vi "Permanent Settings.vi"(11 "Settings in in":T1) -> (3 "Settings out":T1)   [LabVIEW 2013, in "AvaSpec.lvlib" / "AvaSpec Settings.lvlib"]
uses:
  AvaSpec Settings.lvlib
  Settings.ctl
  Acquisition/Hardware Configuration.ctl
  Libraries/AS-5216-DLL/AVS settings.ctl
  Acquisition/Sphere Indicator.ctl
  Measurement Type.ctl
  Logging/Logging Configuration.ctl
  AvaSpec.lvlib
  Acquisition/AvaSpec Acquisition.lvlib
  Logging/AvaSpec Logging.lvlib
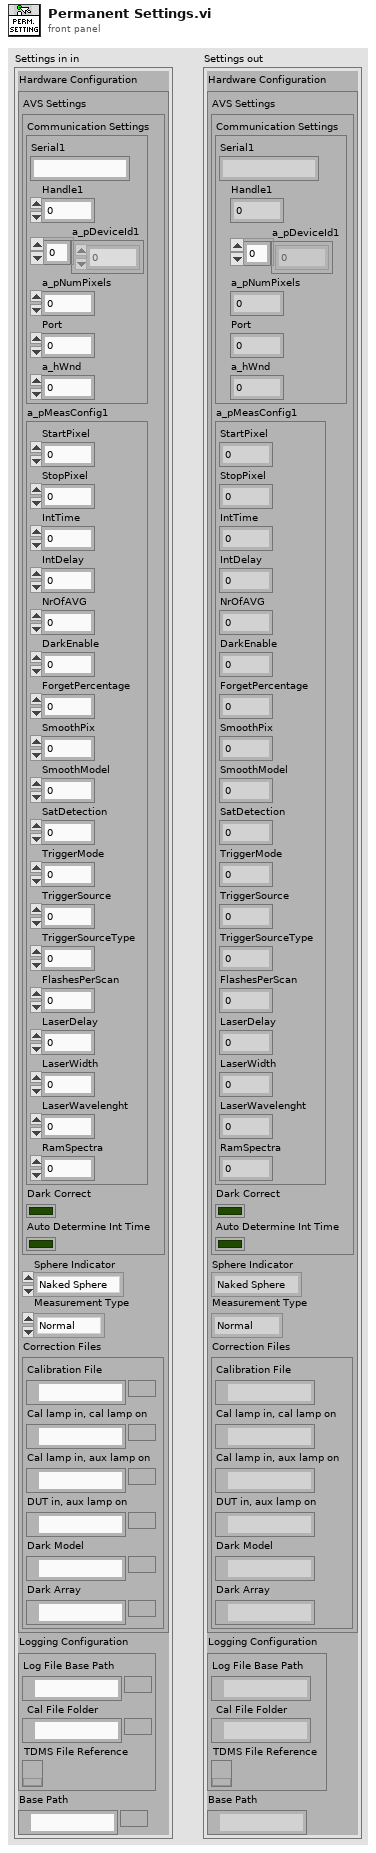
[diagram p1: front panel]
types:
  T1 = typedef "AvaSpec.lvlib/AvaSpec Settings.lvlib/Settings.ctl" = cluster{"Hardware Configuration":T2, "Logging Configuration":T6, "Base Path":path}
  T2 = typedef "AvaSpec.lvlib/AvaSpec Acquisition.lvlib/Hardware Configuration.ctl" = cluster{"AVS Settings":T3, "Sphere Indicator":T4, "Measurement Type":T5, "Correction Files":cluster{"Calibration File":path, "Cal lamp in, cal lamp on":path, "Cal lamp in, aux lamp on":path, "DUT in, aux lamp on":path, "Dark Model":path, "Dark Array":path}}
  T3 = typedef "AvaSpec.lvlib/AVS settings.ctl" = cluster{"Communication Settings":cluster{"Serial1":string, "Handle1":i32, "a_pDeviceId1":u8[], "a_pNumPixels":u16, "Port":i32, "a_hWnd":i32}, "a_pMeasConfig1":cluster{"StartPixel":u16, "StopPixel":u16, "IntTime":sgl, "IntDelay":u32, "NrOfAVG":u32, "DarkEnable":u8, "ForgetPercentage":u8, "SmoothPix":u16, "SmoothModel":u8, "SatDetection":u8, "TriggerMode":u8, "TriggerSource":u8, "TriggerSourceType":u8, "FlashesPerScan":u16, "LaserDelay":u32, "LaserWidth":u32, "LaserWavelenght":sgl, "RamSpectra":u16}, "Dark Correct":bool, "Auto Determine Int Time":bool}
  T4 = typedef "AvaSpec.lvlib/Sphere Indicator.ctl" = enum16{"Naked Sphere", "Insulated Sphere"}
  T5 = typedef "AvaSpec.lvlib/AvaSpec Acquisition.lvlib/Measurement Type.ctl" = enum16{"Normal", "Calibration", "Dark"}
  T6 = typedef "AvaSpec.lvlib/AvaSpec Logging.lvlib/Logging Configuration.ctl" = cluster{"Log File Base Path":path, "Cal File Folder":path, "TDMS File Reference":refnum<k34>}
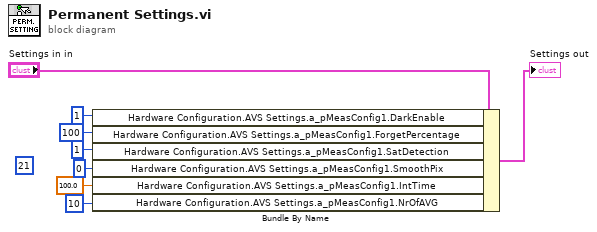
[diagram p0: block diagram]
diagram:
  (unwired) u8 21 ("Hardware Configuration.AVS Settings.a_pMeasConfig1.SmoothModel")
  n1 = Bundle By Name(cluster="Settings in in", "Hardware Configuration.AVS Settings.a_pMeasConfig1.DarkEnable"=u8 1 ("Hardware Configuration.a_pMeasConfig1.DarkEnable"), "Hardware Configuration.AVS Settings.a_pMeasConfig1.ForgetPercentage"=u8 100 ("Hardware Configuration.a_pMeasConfig1.SatDetection"), "Hardware Configuration.AVS Settings.a_pMeasConfig1.SatDetection"=u8 1 ("Hardware Configuration.a_pMeasConfig1.SatDetection"), "Hardware Configuration.AVS Settings.a_pMeasConfig1.SmoothPix"=u16 0, "Hardware Configuration.AVS Settings.a_pMeasConfig1.IntTime"=sgl 100.0, "Hardware Configuration.AVS Settings.a_pMeasConfig1.NrOfAVG"=u32 10) -> (→"Settings out":T1)
